vi "StahlPS_USB.Read_DB.vi"(0 "i ref in":refnum<vi>, 5 "error in (no error)":errorcluster) -> (14 "i ref out":refnum<vi>, 16 "NofChannels":i32, 19 "error out (no error)":errorcluster)   [LabVIEW 2014, in "StahlPS_USB.lvlib"]
doc: "This VI reads outall important Values from the Database (or directly from the Baseprocess Class)"
uses:
  StahlPS_USB.lvlib
  CSCore/BaseProcess/BaseProcess.lvlib
  CSCore/CSSystem/CoreLib/CoreLib.lvlib
  CSCore/CSApplicationBaseClasses/PSChannelBase/PSChannelBase.lvlib
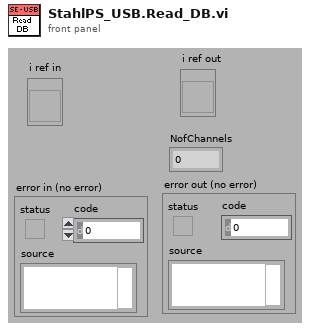
[diagram p1: front panel]
types:
  T1 = typedef "BaseProcess.lvlib/BaseProcess.i attribute.ctl" = cluster{"EventStatus":string, "EventError":i32, "PresetEvtWatchD":i32, "PresetPdcWatchD":i32, "EventTimeout":i32, "PeriodicInterval":i32, "Interface":string[], "Address":string[], "Special":string[], "PeriodicError":i32, "PeriodicStatus":string, "SuperProc":string, "Descriptors":T2[], "CaseRef":refnum<vi>, "PdcRef":refnum<vi>, "Thread Ref":refnum<vi>, "eventErrorID":i32, "eventStatusID":i32, "periodicErrorID":i32, "periodicStatusID":i32, "pdcCtrID":i32}
  T2 = typedef "BaseProcess.lvlib/BaseProcess.descriptor definition.ctl" = cluster{"selector":string, "descriptor":T3}
  T3 = typedef "BaseProcess.lvlib/BaseProcess.descriptor string definition.ctl" = string
  T4 = typedef "StahlPS_USB.lvlib/StahlPS_USB.i attribute.ctl" = cluster{"VISA resource name":refnum<visa-resource-name>, "Type":string, "MaxVoltage":dbl, "MinVoltage":dbl, "Elektrode Names":string[]}
  T5 = typedef "PSChannelBase.lvlib/PSChannelBase.i attribute.ctl" = cluster{"defaultChannelIndex":i32, "nofChannels":i32, "defaultChannelIndexID":i32, "nofChannelsID":i32, "actValues":T6, "nomValues":T6, "logicalName":string[], "physicalName":string[], "logicalNameID":i32, "physicalNameID":i32}
  T6 = typedef "PSChannelBase.lvlib/PSChannelBase.parameters.ctl" = cluster{"onOff":bool[], "voltage":dbl[], "current":dbl[], "tripCurrent":dbl[], "rampUpSpeed":dbl[], "rampDownSpeed":dbl[], "status":i32[], "serviceIDs":cluster{"onOfflID":i32, "voltageID":i32, "currentID":i32, "tripCurrentID":i32, "rampUpSpeedID":i32, "rampDownSpeedID":i32, "statusID":i32}}
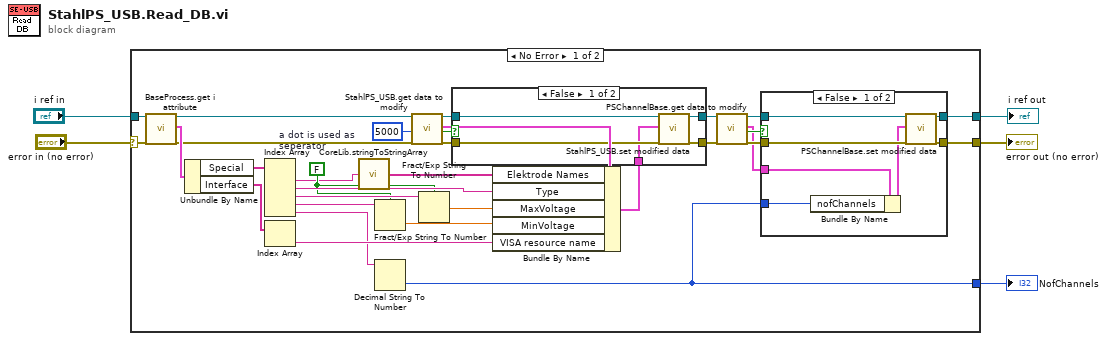
[diagram p0: block diagram]
diagram:
  n1 = case shown="No Error" "error in (no error)" {
    selector: "error in (no error)" -> [w35 w55]
    tunnel: [w10 w55] -> w2
    tunnel: "i ref in" -> [w37 w54]
    tunnel: [w11 w54] -> w4
    tunnel: [w6 _] -> w1
    frame No Error {
      w22 = FALSE  # a dot is used as seperator
      n2 = call "BaseProcess.get i attribute.vi"("i ref in"=w37, "error in (no error)"=w35) -> ("i ref out"=w36:refnum<vi>, "i attribute"=w30:T1, "error out"=w26:errorcluster)  [unwired: 15 in]
      n3 = Unbundle By Name(w30) -> ("Special"=w29:string[], "Interface"=w17:string[])
      n4 = Index Array(array=w29) -> (element #1=w19:string, element #2=w25:string, element #3=w24:string, element #4=w23:string, element #5=w7:string)  [unwired: 5 in]
      n5 = Index Array(array=w17) -> (element=w16:string)  [unwired: 1 in]
      n6 = call "CoreLib.stringToStringArray.vi"("String"=w19) -> ("Array"=w18:string[])
      n7 = Fract/Exp String To Number(use system decimal point (T)=w22, string=w23) -> (number=w31:dbl)  [unwired: 2 in, 1 out]
      n8 = Decimal String To Number(string=w7) -> (number=w6:i32)  [unwired: 2 in, 1 out]
      n9 = call "StahlPS_USB.get data to modify.vi"("i ref in"=w36, "ms timeout (10000)"=5000, "error in (no error)"=w26) -> ("i ref out"=w34:refnum<vi>, "i attribute"=w28:T4, "timed out"=w21:bool, "error out"=w33:errorcluster)  [unwired: 13 in]
      n10 = Fract/Exp String To Number(use system decimal point (T)=w22, string=w24) -> (number=w32:dbl)  [unwired: 2 in, 1 out]
      n11 = Bundle By Name(cluster=w28, "Elektrode Names"=w18, "Type"=w25, "MaxVoltage"=w32, "MinVoltage"=w31, "VISA resource name"=w16) -> (w27:T4)
      n12 = case shown="False" w21 {
        tunnel: [w51 w53] -> w14
        tunnel: [w50 w52] -> w15
        tunnel: w34 -> [w49 w53]
        tunnel: w33 -> [w48 w52]
        tunnel: w27 -> [w47 _]
        frame False {
          n13 = call "StahlPS_USB.set modified data.vi"("i ref in"=w49, "i attribute"=w47, "error in (no error)"=w48) -> ("i ref out"=w51:refnum<vi>, "error out"=w50:errorcluster)  [unwired: 15 in]
        }
        frame True {
        }
      }
      n14 = call "PSChannelBase.get data to modify.vi"("i ref in"=w14, "error in (no error)"=w15) -> ("i ref out"=w13:refnum<vi>, "i attribute"=w8:T5, "timed out"=w9:bool, "error out"=w12:errorcluster)  [unwired: 14 in]
      n15 = case shown="False" w9 {
        tunnel: w13 -> [w44 w46]
        tunnel: w12 -> [w43 w45]
        tunnel: [w42 w46] -> w11
        tunnel: [w41 w45] -> w10
        tunnel: w8 -> [w40 _]
        tunnel: w6 -> [w38 _]
        frame False {
          n16 = Bundle By Name(cluster=w40, "nofChannels"=w38) -> (w39:T5)
          n17 = call "PSChannelBase.set modified data.vi"("i ref in"=w44, "i attribute"=w39, "error in (no error)"=w43) -> ("i ref out"=w42:refnum<vi>, "error out"=w41:errorcluster)  [unwired: 15 in]
        }
        frame True {
        }
      }
    }
    frame Error {
    }
  }
  "error out (no error)" <- w2
  "i ref out" <- w4
  "NofChannels" <- w1
